vi "Lab8_front_panel.vi"() -> ()   [LabVIEW 2024]
uses:
  <vilib>/Utility/error.llb/Trim Whitespace One-Sided.vi
  <vilib>/Instr/_visa.llb/VISA Configure Serial Port (Instr).vi
  <vilib>/Analysis/NI_AALPro.lvlib
panel:
  out "ADC NL":cluster{"Best Exponential Fit":dbl[], dbl[]}(graph)
  in  "Medie":bool
  out "Offset":dbl
  out "C [pF]":dbl
  in  "dT":dbl
  out "Residui":cluster{dbl[], dbl[]}(graph)
  out "Segnale":cluster{"Best Exponential Fit":dbl[], dbl[]}[](graph)
  in  "Stop":bool
  in  "Lenght":dbl
  in  "Begin":dbl
  in  "Porta VISA":refnum<visa-resource-name>
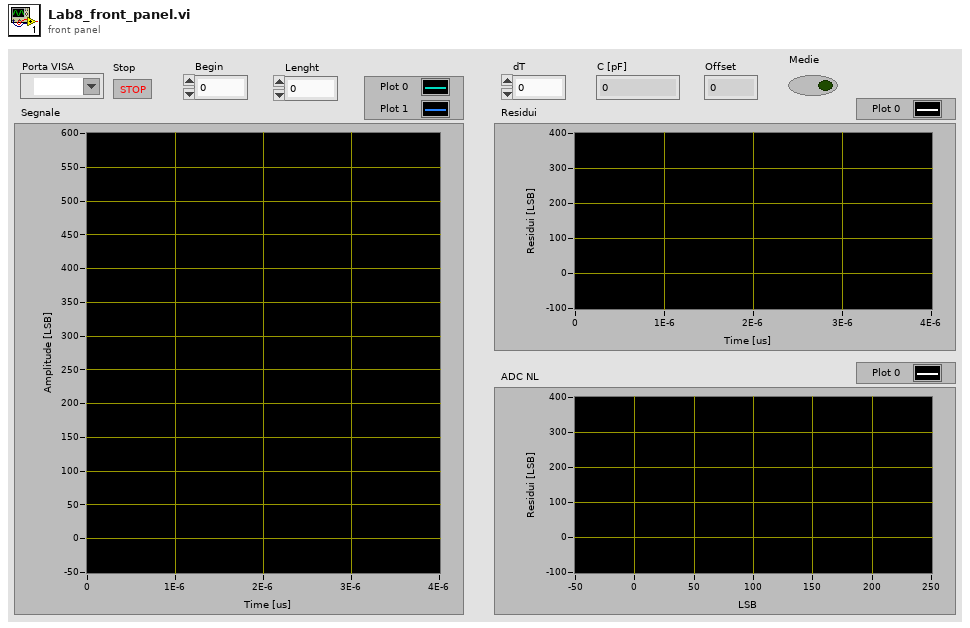
[diagram p1: front panel]
types:
  T1 = enum16{"open", "replace", "create", "open or create", "replace or create", "replace or create with confirmation"}
  T2 = cluster{"amp min":dbl, "amp max":dbl, "damping min":dbl, "damping max":dbl, "offset min":dbl, "offset max":dbl}
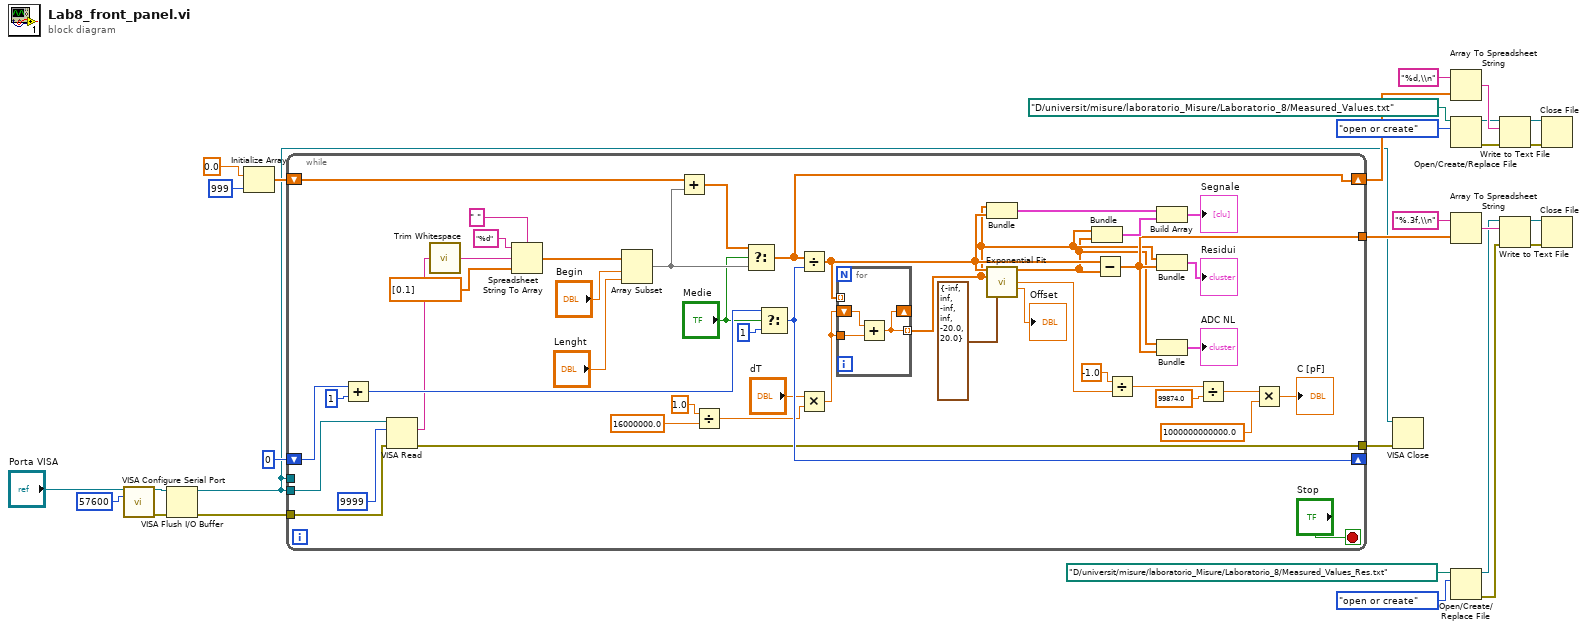
[diagram p0: block diagram]
diagram:
  n1 = call-poly "VISA Configure Serial Port"("VISA resource name"="Porta VISA", "baud rate (9600)"=u32 57600) -> ("VISA resource name out"=w20:refnum<visa-resource-name>, "error out"=w27:errorcluster)  [unwired: 12 in]
  n2 = VISA Flush I/O Buffer(VISA resource name=w20, error in (no error)=w27) -> (VISA resource name out=w1:refnum<visa-resource-name>, error out=w26:errorcluster)  [unwired: 1 in]
  n3 = Initialize Array(0.0 ("element"), 999 ("dimension size")) -> (w22:dbl[])
  n4 = while {
    tunnel: w1 -> [w75]
    tunnel: w26 -> [w74]
    shift-right: [w57] -> _
    shift-left: u32 0 ("byte count") -> [w65]
    shift-right: [w56] -> w16
    shift-left: w22 -> [w61]
    tunnel: [w35] -> w21
    tunnel: [w36] -> w3
    tunnel: w1 -> [_]
    stop <- "Stop" stop-if-true
    n5 = Add(x=w65, y=u32 1) -> (x+y=w63:u32)
    n6 = VISA Read(VISA resource name=w75, byte count=u32 9999, error in (no error)=w74) -> (read buffer=w33:string, error out=w35:errorcluster)  [unwired: 2 out]
    n7 = call <vilib>:"Trim Whitespace.vi"("string"=w33) -> ("trimmed string"=w71:string)  [unwired: 1 in]
    n8 = Spreadsheet String To Array(delimiter (Tab)=" ", format string="%d", spreadsheet string=w71, array type (2D Dbl)=dbl[] [0.1]) -> (array=w68:dbl[])
    n9 = Array Subset(array=w68, index="Begin", length="Lenght") -> (w60:dbl[])
    n10 = Add(x=w61, y=w60) -> (x+y=w59:dbl[])
    n11 = Divide(x=1.0, y=16000000.0) -> (x/y=w50:dbl)
    n12 = Select(t=w59, s="Medie", f=w60) -> (s? t:f=w56:dbl[])
    n13 = Select(t=w63, s="Medie", f=u32 1) -> (s? t:f=w57:u32)
    n14 = Divide(x=w56, y=w57) -> (x/y=w32:dbl[])
    n15 = Multiply(x="dT", y=w50) -> (x*y=w49:dbl)
    n16 = for {
      tunnel: w32 -> [_] mode=indexing
      shift-right: [w76] -> _
      shift-left: w49 -> [w78]
      tunnel: w49 -> [w77]
      tunnel: [w76] -> w31 mode=indexing
      n17 = Add(x=w78, y=w77) -> (x+y=w76:dbl)
    }
    n18 = Bundle(w31, w32) -> (w41:cluster{dbl[], dbl[]})  [unwired: 1 in]
    n19 = call <vilib>:"Exponential Fit.vi"("Y"=w32, "X"=w31, "parameter bounds"=T2 {"amp min"=-inf, "amp max"=inf, "damping min"=-inf, "damping max"=inf, "offset min"=-20.0, "offset max"=20.0}) -> ("Best Exponential Fit"=w30:dbl[], "damping"=w47:dbl, "offset"=→"Offset":dbl)  [unwired: 7 in, 3 out]
    n20 = Bundle(w31, "Best Exponential Fit"=w30) -> (w40:cluster{dbl[], "Best Exponential Fit":dbl[]})  [unwired: 1 in]
    n21 = Subtract(x=w32, y=w30) -> (x-y=w36:dbl[])
    n22 = Divide(x=-1.0, y=w47) -> (x/y=w46:dbl)
    n23 = Build Array(w41, w40) -> (→"Segnale":cluster{dbl[], "Best Exponential Fit":dbl[]}[])
    n24 = Bundle(w31, w36) -> (→"Residui":cluster{dbl[], dbl[]})  [unwired: 1 in]
    n25 = Bundle("Best Exponential Fit"=w30, w36) -> (→"ADC NL":cluster{"Best Exponential Fit":dbl[], dbl[]})  [unwired: 1 in]
    n26 = Divide(x=w46, y=99874.0) -> (x/y=w44:dbl)
    n27 = Multiply(x=w44, y=1000000000000.0) -> (x*y=→"C [pF]":dbl)
  }
  n28 = VISA Close(VISA resource name=w1, error in (no error)=w21) -> ()  [unwired: 1 out]
  n29 = Array To Spreadsheet String(array=w16, 3:"%d,\\n" ("format string")) -> (spreadsheet string=w15:string)  [unwired: 1 in]
  n30 = Open/Create/Replace File(file path (use dialog)=path "D:/universit/misure/laboratorio_Misure/Laboratorio_8/Measured_Values.txt", operation (0:open)=T1."open or create") -> (refnum out=w14:refnum<file>, error out=w13:errorcluster)  [unwired: 4 in, 1 out]
  n31 = Array To Spreadsheet String(array=w3, 3:"%.3f,\\n" ("format string")) -> (spreadsheet string=w8:string)  [unwired: 1 in]
  n32 = Open/Create/Replace File(file path (use dialog)=path "D:/universit/misure/laboratorio_Misure/Laboratorio_8/Measured_Values_Res.txt", operation (0:open)=T1."open or create") -> (refnum out=w7:refnum<file>, error out=w6:errorcluster)  [unwired: 4 in, 1 out]
  n33 = Write to Text File(file (use dialog)=w14, text=w15, error in=w13) -> (refnum out=w11:refnum<file>, error out=w12:errorcluster)  [unwired: 1 in, 1 out]
  n34 = Write to Text File(file (use dialog)=w7, text=w8, error in=w6) -> (refnum out=w4:refnum<file>, error out=w5:errorcluster)  [unwired: 1 in, 1 out]
  n35 = Close File(refnum=w11, error in=w12) -> ()  [unwired: 2 out]
  n36 = Close File(refnum=w4, error in=w5) -> ()  [unwired: 2 out]
